vi "PORT IO Enable Range__ogtk.vi"(4 "error in (no error)":errorcluster, 6 "size":u16, 7 "start address":u16 format="%.0x") -> (0 "error out":errorcluster)   [LabVIEW 2012]
doc: "This function enables user space access to a range of IO ports for the current process. This function has no effect on Windows 95/98/ME based operating systems."
uses:
  <userlib>/_OpenG.lib/portio/ogportio.dll
panel:
  # "[OpenG VI Tags] ***Do Not Remove***"
  # "PORT IO Enable Range.vi\n\nEnables a range of IO addresses to be accessed directly from user space.\n\nPlease visit http://www.OpenG.org to learn about the\nOpen Source LabVIEW software movement.\n\nNOTICE -- YOU MUST LEAVE THIS NOTICE IN PLACE.  PER THE TERMS OF THE LICENSE BELOW, YOU MAY SUBLICENSE THIS SOFTWARE \nIN ANY WAY THAT DOES NOT CONFLICT WITH THIS LICENSE.\n\n### BSD License (http://www.opensource.org/licenses/bsd-license.php) Begin ###\n\nCopyright (c) 2002-2007, Rolf Kalbermatter <rolf.kalbermatter@citeng.com> \n\nAll rights reserved.\n\nRedistribution and use in source and binary forms, with or without modification, are permitted provided that the following conditions are met:\n\n    * Redistributions of source code must retain the above copyright notice, this list of conditions and the following disclaimer.\n    * Redistributions in binary form must reproduce the above copyright notice, this list of conditions and the following disclaimer in the \n       documentation and/or other materials provided with the distribution.\n    * Neither the name of SciWare, James Kring, Inc., nor the names of its contributors may be used to endorse or promote products derived \n       from this software without specific prior written permission.\n\nTHIS SOFTWARE IS PROVIDED BY THE COPYRIGHT HOLDERS AND CONTRIBUTORS \"AS IS\" AND ANY EXPRESS OR IMPLIED WARRANTIES, \nINCLUDING, BUT NOT LIMITED TO, THE IMPLIED WARRANTIES OF MERCHANTABILITY AND FITNESS FOR A PARTICULAR PURPOSE ARE \nDISCLAIMED. IN NO EVENT SHALL THE COPYRIGHT OWNER OR CONTRIBUTORS BE LIABLE FOR ANY DIRECT, INDIRECT, INCIDENTAL,\n SPECIAL, EXEMPLARY, OR CONSEQUENTIAL DAMAGES (INCLUDING, BUT NOT LIMITED TO, PROCUREMENT OF SUBSTITUTE GOODS OR \nSERVICES; LOSS OF USE, DATA, OR PROFITS; OR BUSINESS INTERRUPTION) HOWEVER CAUSED AND ON ANY THEORY OF LIABILITY, \nWHETHER IN CONTRACT, STRICT LIABILITY, OR TORT (INCLUDING NEGLIGENCE OR OTHERWISE) ARISING IN ANY WAY OUT OF THE USE \nOF THIS SOFTWARE, EVEN IF ADVISED OF THE POSSIBILITY OF SUCH DAMAGE.\n\n### BSD License End ###"
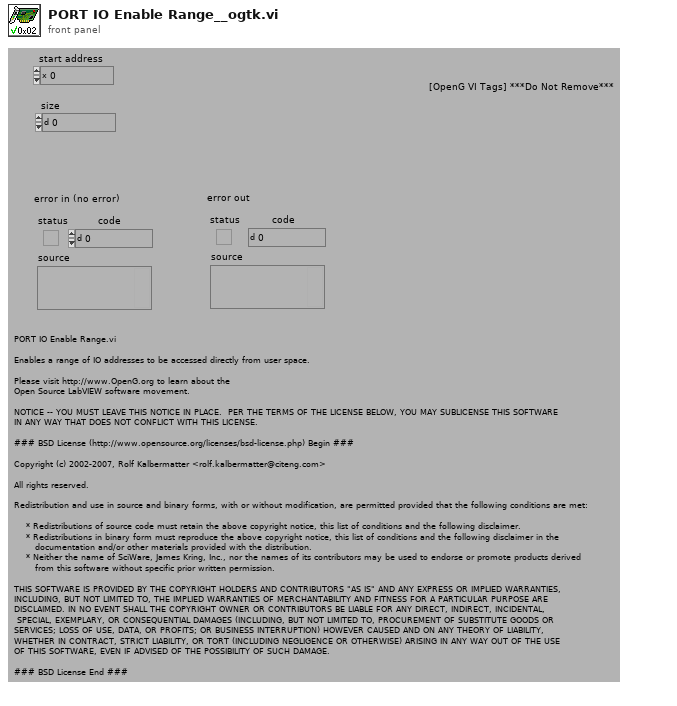
[diagram p1: front panel]
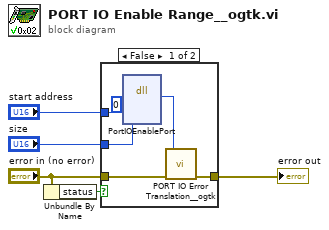
[diagram p0: block diagram]
diagram:
  n1 = Unbundle By Name("error in (no error)") -> ("status"=w5:bool)
  n2 = case shown="False" w5 {
    tunnel: [w6 w12] -> w3
    tunnel: "error in (no error)" -> [w7 w12]
    tunnel: "start address" -> [w11 _]
    tunnel: "size" -> [w10 _]
    frame False {
      n3 = dll-call lib="C:/Program Files/National Instruments/LabVIEW 2012/user.lib/_OpenG.lib/portio/ogportio.*" fn="PortIOEnablePort"("process"=u32 0, "start"=w11, "size"=w10) -> (w8:u32)  [unwired: 6 in, 2 out]
      n4 = call <userlib>:"PORT IO Error Translation__ogtk.vi"("error in (no error)"=w7, "win error"=w8) -> ("error out"=w6:errorcluster)  [unwired: 5 in]
    }
    frame True {
      (unwired) u32 0
    }
  }
  "error out" <- w3
